vi "ExcelUnitTest.vi"() -> ()   [LabVIEW 2015, in "Excel.lvclass"]
uses:
  Excel.lvclass
panel:
  out "Data":string[][](array[string])
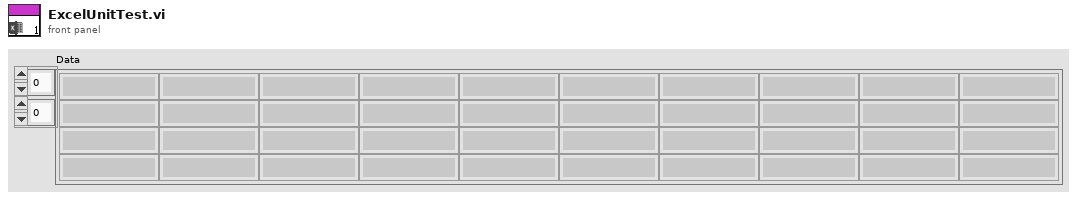
[diagram p1: front panel]
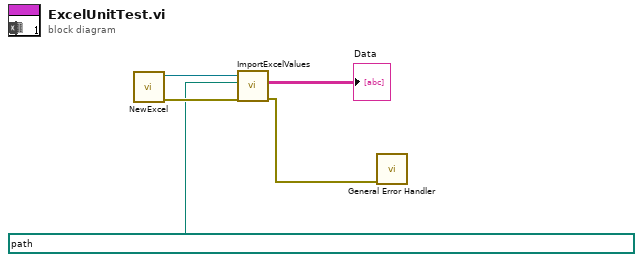
[diagram p0: block diagram]
diagram:
  n1 = call "NewExcel.vi"() -> ("error out"=w4:errorcluster, "Excel out"=w5:refnum<class "Excel.lvclass">)  [unwired: 10 in]
  n2 = call "ImportExcelValues.vi"("error in (no error)"=w4, "ExcelPath"=path "E:/LabVIEW相关/LabVIEW项目/机电学院档案管理系统_201603/LV/Archive/resources/_excel/学籍档案模板.xlsx", "Excel in"=w5) -> ("error out"=w1:errorcluster, "Data"=→"Data":string[][])  [unwired: 6 in, 1 out]
  n3 = call <vilib>:"General Error Handler.vi"("error in (no error)"=w1) -> ()  [unwired: 10 in, 5 out]
